vi "GEOM_CheckFullROI.vi"(6 "self":bool=TRUE, 9 "amproi":T1={"xstart"=1, "ystart"=1, "xsize"=1, "ysize"=1}, 10 "Amplifier":T2 {"fliped" items=["none", "horizontal", "vertical"]; "type" items=["LL", "LR", "UL", "UR"]}) -> (2 "full":bool)   [LabVIEW 2016]
uses:
  GEOM_Amplifier.ctl
  GEOM_AmpType.ctl
  GEOM_ROI.ctl
  GEOM_Coords.ctl
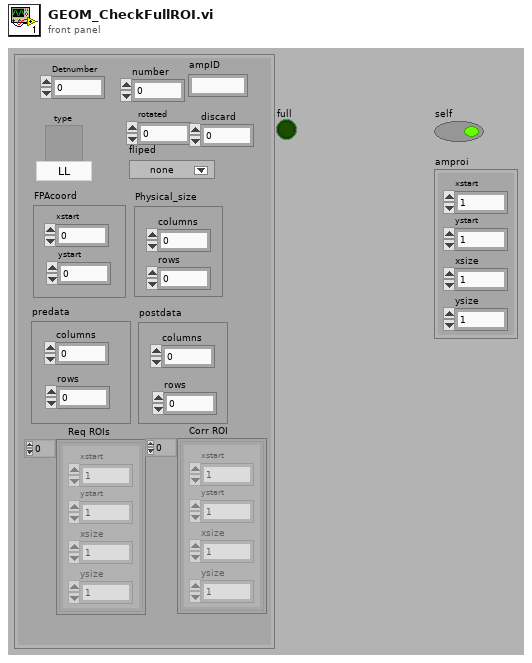
[diagram p1: front panel]
types:
  T1 = typedef "GEOM_Coords.ctl" = cluster{"xstart":u32, "ystart":u32, "xsize":u32, "ysize":u32}
  T2 = typedef "GEOM_Amplifier.ctl" = cluster{"number":i32, "type":T3, "rotated":i16, "fliped":u16, "FPAcoord":cluster{"xstart":i32, "ystart":i32}, "Physical_size":cluster{"columns":i32, "rows":i32}, "predata":cluster{"columns":i32, "rows":i32}, "postdata":cluster{"columns":i32, "rows":i32}, "Req ROIs":T4, "Corr ROI":T4, "Detnumber":i32, "ampID":string, "discard":i32}
  T3 = typedef "GEOM_AmpType.ctl" = u16
  T4 = typedef "GEOM_ROI.ctl" = T1[]
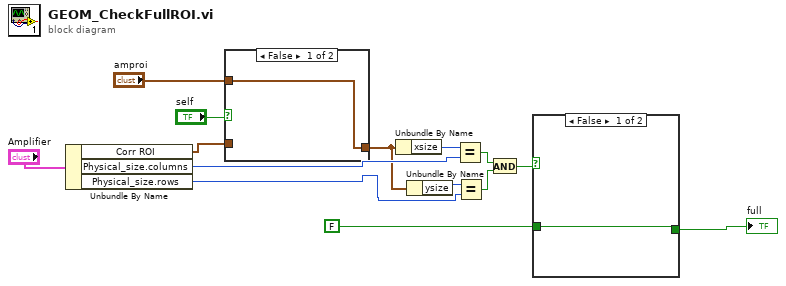
[diagram p0: block diagram]
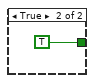
[diagram p2: hidden frame]
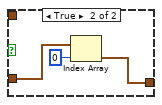
[diagram p3: hidden frame]
diagram:
  n1 = Unbundle By Name("Amplifier") -> ("Corr ROI"=w9:T4, "Physical_size.columns"=w13:i32, "Physical_size.rows"=w12:i32)
  n2 = case shown="False" "self" {
    tunnel: w9 -> [_ w18]
    tunnel: [w15 w16] -> w3
    tunnel: "amproi" -> [w15 _]
    frame False {
    }
    frame True {
      n3 = Index Array(array=w18, index=0) -> (element=w16:T1)
    }
  }
  n4 = Unbundle By Name(w3) -> ("xsize"=w1:u32)
  n5 = Unbundle By Name(w3) -> ("ysize"=w2:u32)
  n6 = Equal?(x=w1, y=w13) -> (x = y?=w7:bool)
  n7 = Equal?(x=w2, y=w12) -> (x = y?=w6:bool)
  n8 = And(x=w7, y=w6) -> (x .and. y?=w5:bool)
  n9 = case shown="False" w5 {
    tunnel: [w19 TRUE] -> w10
    tunnel: FALSE -> [w19 _]
    frame False {
    }
    frame True {
    }
  }
  "full" <- w10
